vi "ContMeas_Label Localization.vi"() -> (2 "localized control labels":string[](array[string]), 3 "DNL_unlocalized control labels":string[](array[string]), 4 "DNL_unlocalized string constant labels":string[](array[string]), 6 "localized string constant values":string[](array[string]))   [LabVIEW 2022 SP3]
panel:
  in  "static localized string constant values":string[](array[string])=["The invalid message string \"%s\" was received in the Acquisition Loop.", "LVM File", "The invalid message string \"%s\" was received in the Logging Loop.", "Exit", "Ready...", "Waiting for trigger", "The invalid message string \"%s\" was received in the Message Handling Loop.", "Logging", "Are you sure you want to quit while the acquisition is running?", "Yes", "No"]
  in  "static localized control labels":string[](array[string])
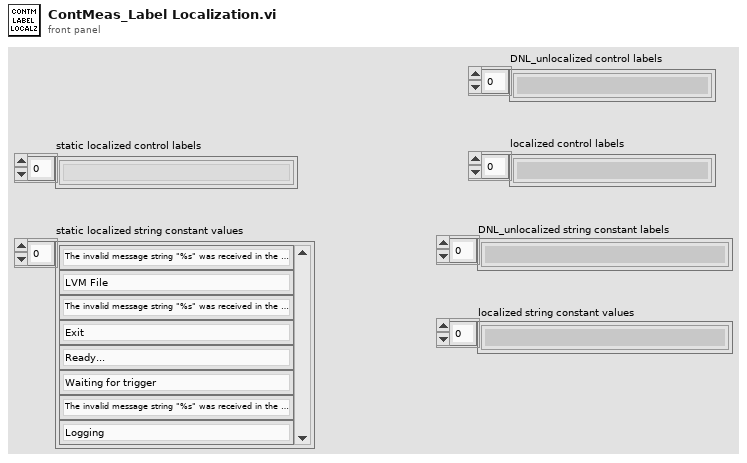
[diagram p1: front panel]
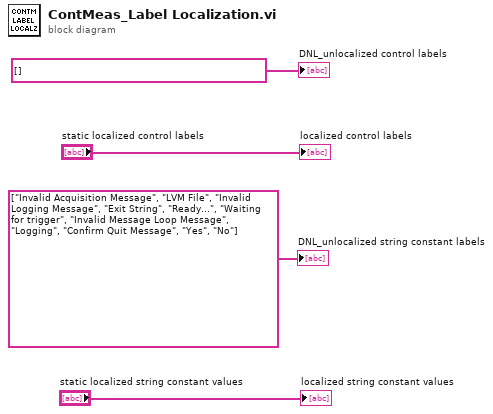
[diagram p0: block diagram]
diagram:
  "DNL_unlocalized control labels" <- string[] [] ("DNL_unlocalized control labels")
  "localized control labels" <- "static localized control labels"
  "localized string constant values" <- "static localized string constant values"
  "DNL_unlocalized string constant labels" <- string[] ["Invalid Acquisition Message", "LVM File", "Invalid Logging Message", "Exit String", "Ready...", "Waiting for trigger", "Invalid Message Loop Message", "Logging", "Confirm Quit Message", "Yes", "No"] ("DNL_unlocalized control labels")
